vi "oscilloscopes_Acquire_Multiple_Waveforms.vi"(3 "error in (no error)":errorcluster, 4 "Channels":i32[](array[ring]) items=["Channel 1"=0, "Channel 2"=1, "Channel 3"=2, "Channel 4"=3, "Waveform Memory 1"=5, "Waveform Memory 2"=6, "Serial Bus 1"=7, "Serial Bus 2"=8, "Digital Bus Low"=9, "Digital Bus High "=10, "Digital Bus 1"=11, "Digital Bus 2"=12, "Function 1"=32, "Function 2"=33, "Function 3"=34, "Function 4"=35, "Math 1"=36, "Math 2"=37, "Math 3"=38, "Math 4"=39], 5 "VISA resource name":refnum<visa-resource-name>) -> (0 "error out":errorcluster, 1 "VISA resource name out":refnum<visa-resource-name>, 2 "Y":dbl[][](array[numeric]))   [LabVIEW 2018]
doc: "This example shows how to configure multiple channels and acquire waveforms from multiple channels."
uses:
  <instrlib>/Agilent 2000 3000 X-Series/Agilent 2000 3000 X-Series.lvlib
panel:
  out "Waveform Data":waveform(dbl)[](graph)
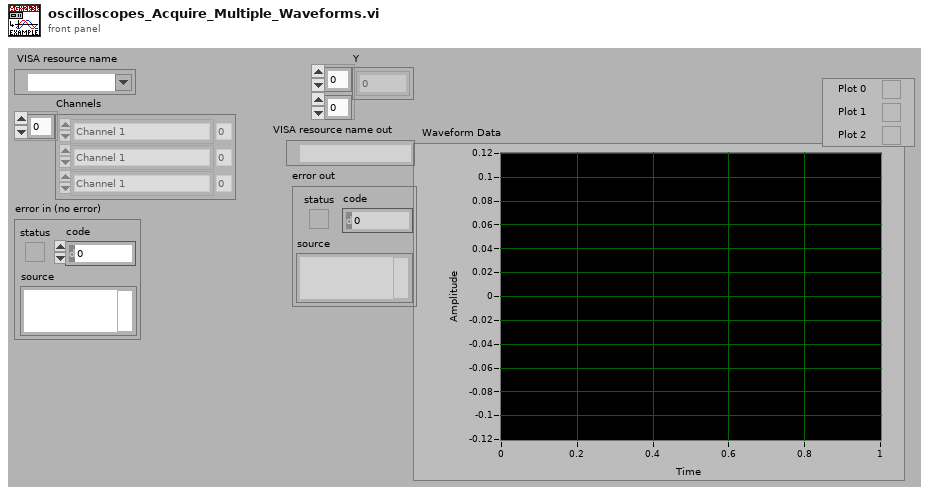
[diagram p1: front panel]
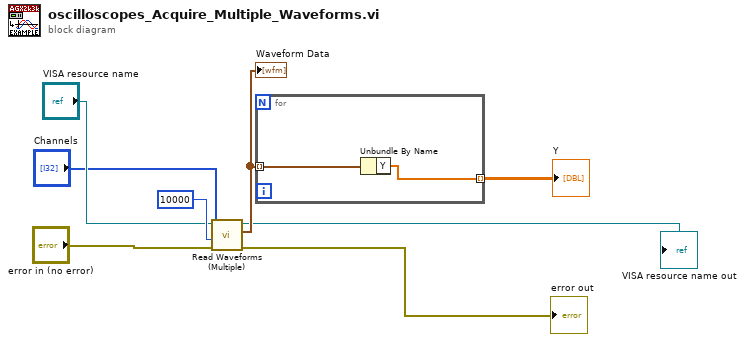
[diagram p0: block diagram]
diagram:
  n1 = call <instrlib>:"Read Waveforms (Multiple).vi"("error in (no error)"="error in (no error)", "Timeout (10000 ms)"=u32 10000 ("Maximum Time (10000 ms)"), "Channels"="Channels", "VISA resource name"="VISA resource name") -> ("error out"=→"error out":errorcluster, "Waveform Data"=w7:waveform(dbl)[], "VISA resource name out"=→"VISA resource name out":refnum<visa-resource-name>)  [unwired: 5 out]
  "Waveform Data" <- w7
  n2 = for {
    tunnel: w7 -> [w10] mode=indexing
    tunnel: [w9] -> w6 mode=indexing
    n3 = Unbundle By Name(w10) -> ("Y"=w9:dbl[])
  }
  "Y" <- w6
